vi "System3.vi"() -> ()   [LabVIEW 2015]
uses:
  <vilib>/addons/control/pid/NI_PID_autopid.lvlib
  <vilib>/DAQmx/write.llb/DAQmx Write (Analog DBL 1Chan 1Samp).vi
  <vilib>/DAQmx/read.llb/DAQmx Read (Analog 1D Wfm NChan NSamp).vi
  <vilib>/Analysis/NI_AALBase.lvlib
  <vilib>/Analysis/baseanly.llb/Mean (DBL).vi
  <vilib>/DAQmx/write.llb/DAQmx Write (Digital 1D Bool NChan 1Samp 1Line).vi
  Control 1.ctl
panel:
  in  "Open/Close (Green)":bool
  in  "Open/Close (Blue)":bool
  in  "Stop program":bool
  in  "On/Off":bool
  in  "Manual Control 2":bool
  in  "Voltage setting 2":dbl format="%#_13g"
  out "Voltage Reading(pressure) 2":dbl format="%#_13g"
  out "Pressure 2":dbl format="%#.3g"
  out "Pressure Chart 2":dbl(graph)
  in  "autotuning parameters 2":T1={"controller type"=1, "relay cycles"=3, "relay amplitude"=1.0, "control specification"=2, "PV noise level"=0.1} {"PV noise level" format="%.2f"; "control specification" items=["normal", "fast", "slow"]; "relay amplitude" format="%.2f"; "controller type" items=["PID", "PI", "P"]}
  in  "PID gains 2":T2={"proportional gain (Kc)"=1.0, "integral time (Ti, min)"=0.01, "derivative time (Td, min)"=0.0} {"derivative time (Td, min)" format="%.3f"; "integral time (Ti, min)" format="%.3f"; "proportional gain (Kc)" format="%.3f"}
  out "PID gains out 2":T2={"proportional gain (Kc)"=1.0, "integral time (Ti, min)"=0.01, "derivative time (Td, min)"=0.0} {"derivative time (Td, min)" format="%.3f"; "integral time (Ti, min)" format="%.3f"; "proportional gain (Kc)" format="%.3f"}
  in  "autotune? (F) 2":bool
  in  "reinitialize? (F) 2":bool
  in  "setpoint in Bar 2":dbl format="%#.5f"
  out "Control Value 2":dbl
  in  "Voltage setting":dbl format="%#_13g"
  in  "Manual Control":bool
  out "Control Value":dbl
  in  "setpoint in Bar":dbl format="%#.5f"
  in  "reinitialize? (F)":bool
  in  "autotune? (F)":bool
  out "PID gains out":T2={"proportional gain (Kc)"=1.0, "integral time (Ti, min)"=0.01, "derivative time (Td, min)"=0.0} {"derivative time (Td, min)" format="%.3f"; "integral time (Ti, min)" format="%.3f"; "proportional gain (Kc)" format="%.3f"}
  in  "PID gains":T2={"proportional gain (Kc)"=1.0, "integral time (Ti, min)"=0.01, "derivative time (Td, min)"=0.0} {"derivative time (Td, min)" format="%.3f"; "integral time (Ti, min)" format="%.3f"; "proportional gain (Kc)" format="%.3f"}
  in  "autotuning parameters":T1={"controller type"=1, "relay cycles"=3, "relay amplitude"=1.0, "control specification"=2, "PV noise level"=0.1} {"PV noise level" format="%.2f"; "control specification" items=["normal", "fast", "slow"]; "relay amplitude" format="%.2f"; "controller type" items=["PID", "PI", "P"]}
  out "Pressure Chart":dbl(graph)
  out "Pressure":dbl format="%#.3g"
  out "Voltage Reading(pressure)":dbl format="%#_13g"
  # "Pressure Vessel 2"
  # "Pressure Vessel 1"
  # "Readings"
  # "Controls"
  # "Readings"
  # "Controls"
  # "PID Settings"
  # "51.12139\n\n0.044676"
  # "Valves"
  # "Pump 3"
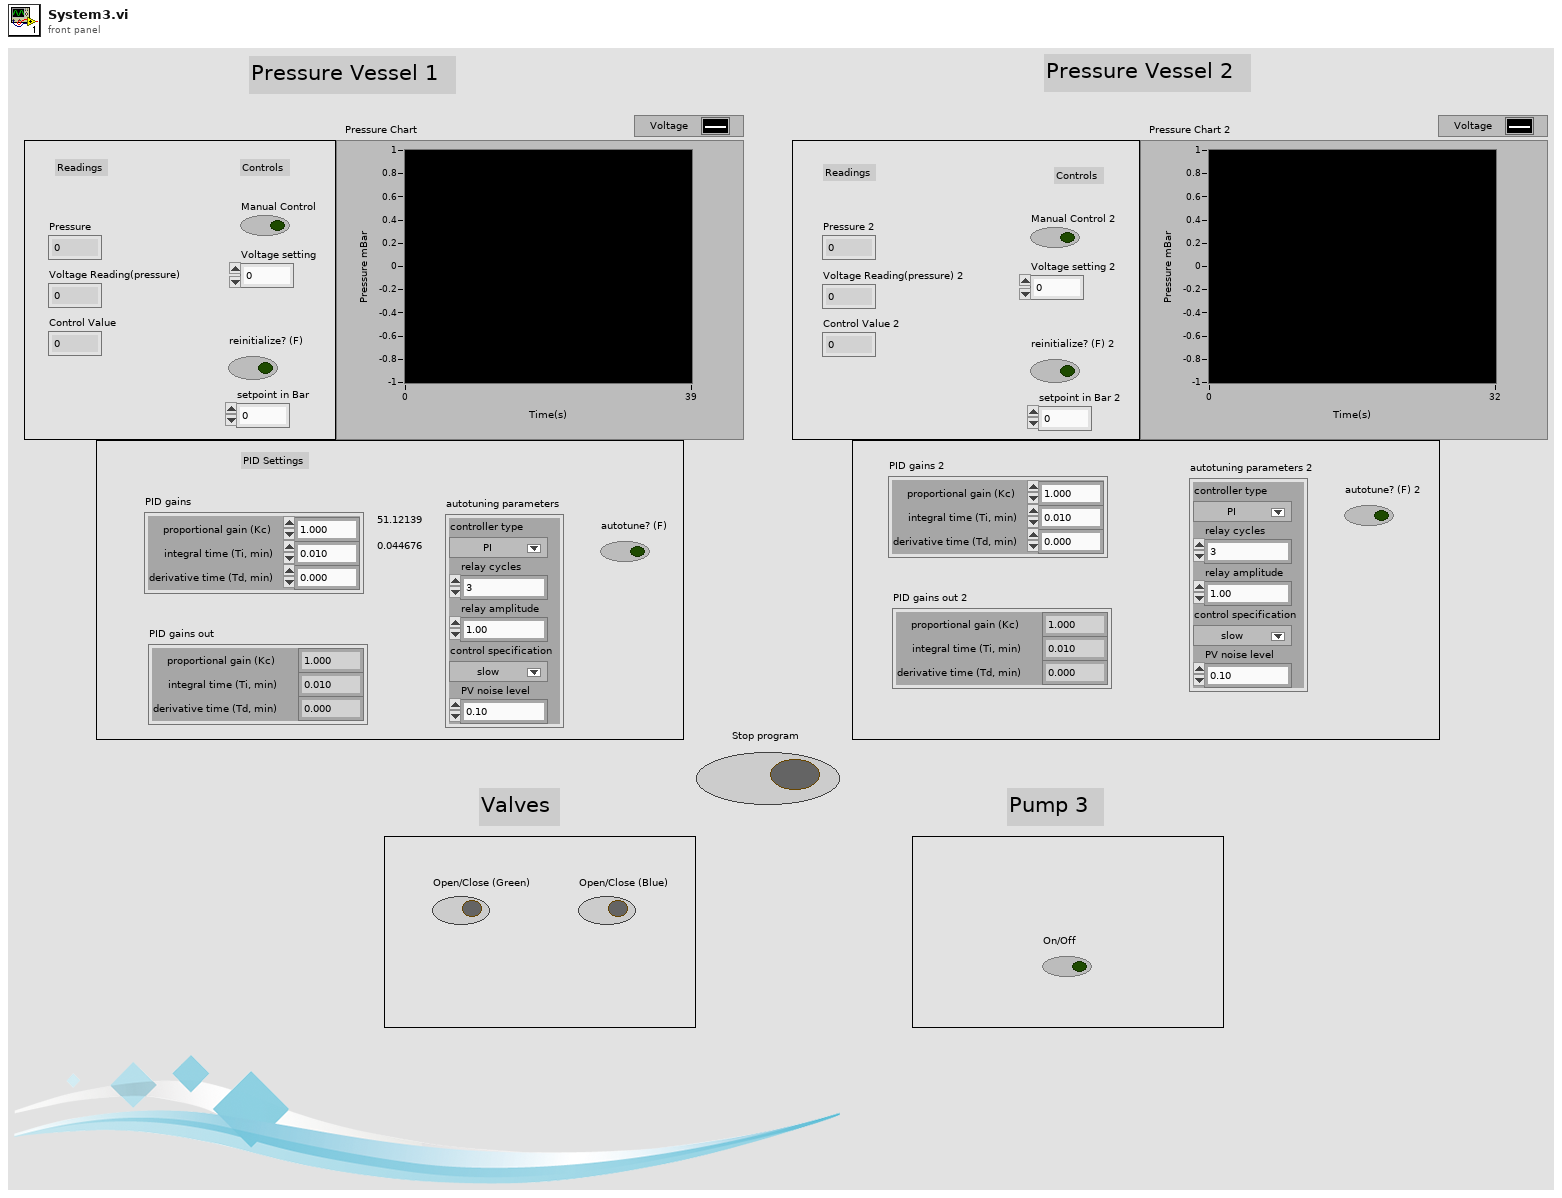
[diagram p1: front panel]
types:
  T1 = cluster{"controller type":u16, "relay cycles":i32, "relay amplitude":dbl, "control specification":u16, "PV noise level":dbl}
  T2 = cluster{"proportional gain (Kc)":dbl, "integral time (Ti, min)":dbl, "derivative time (Td, min)":dbl}
  T3 = typedef "Control 1.ctl" = refnum<k21>
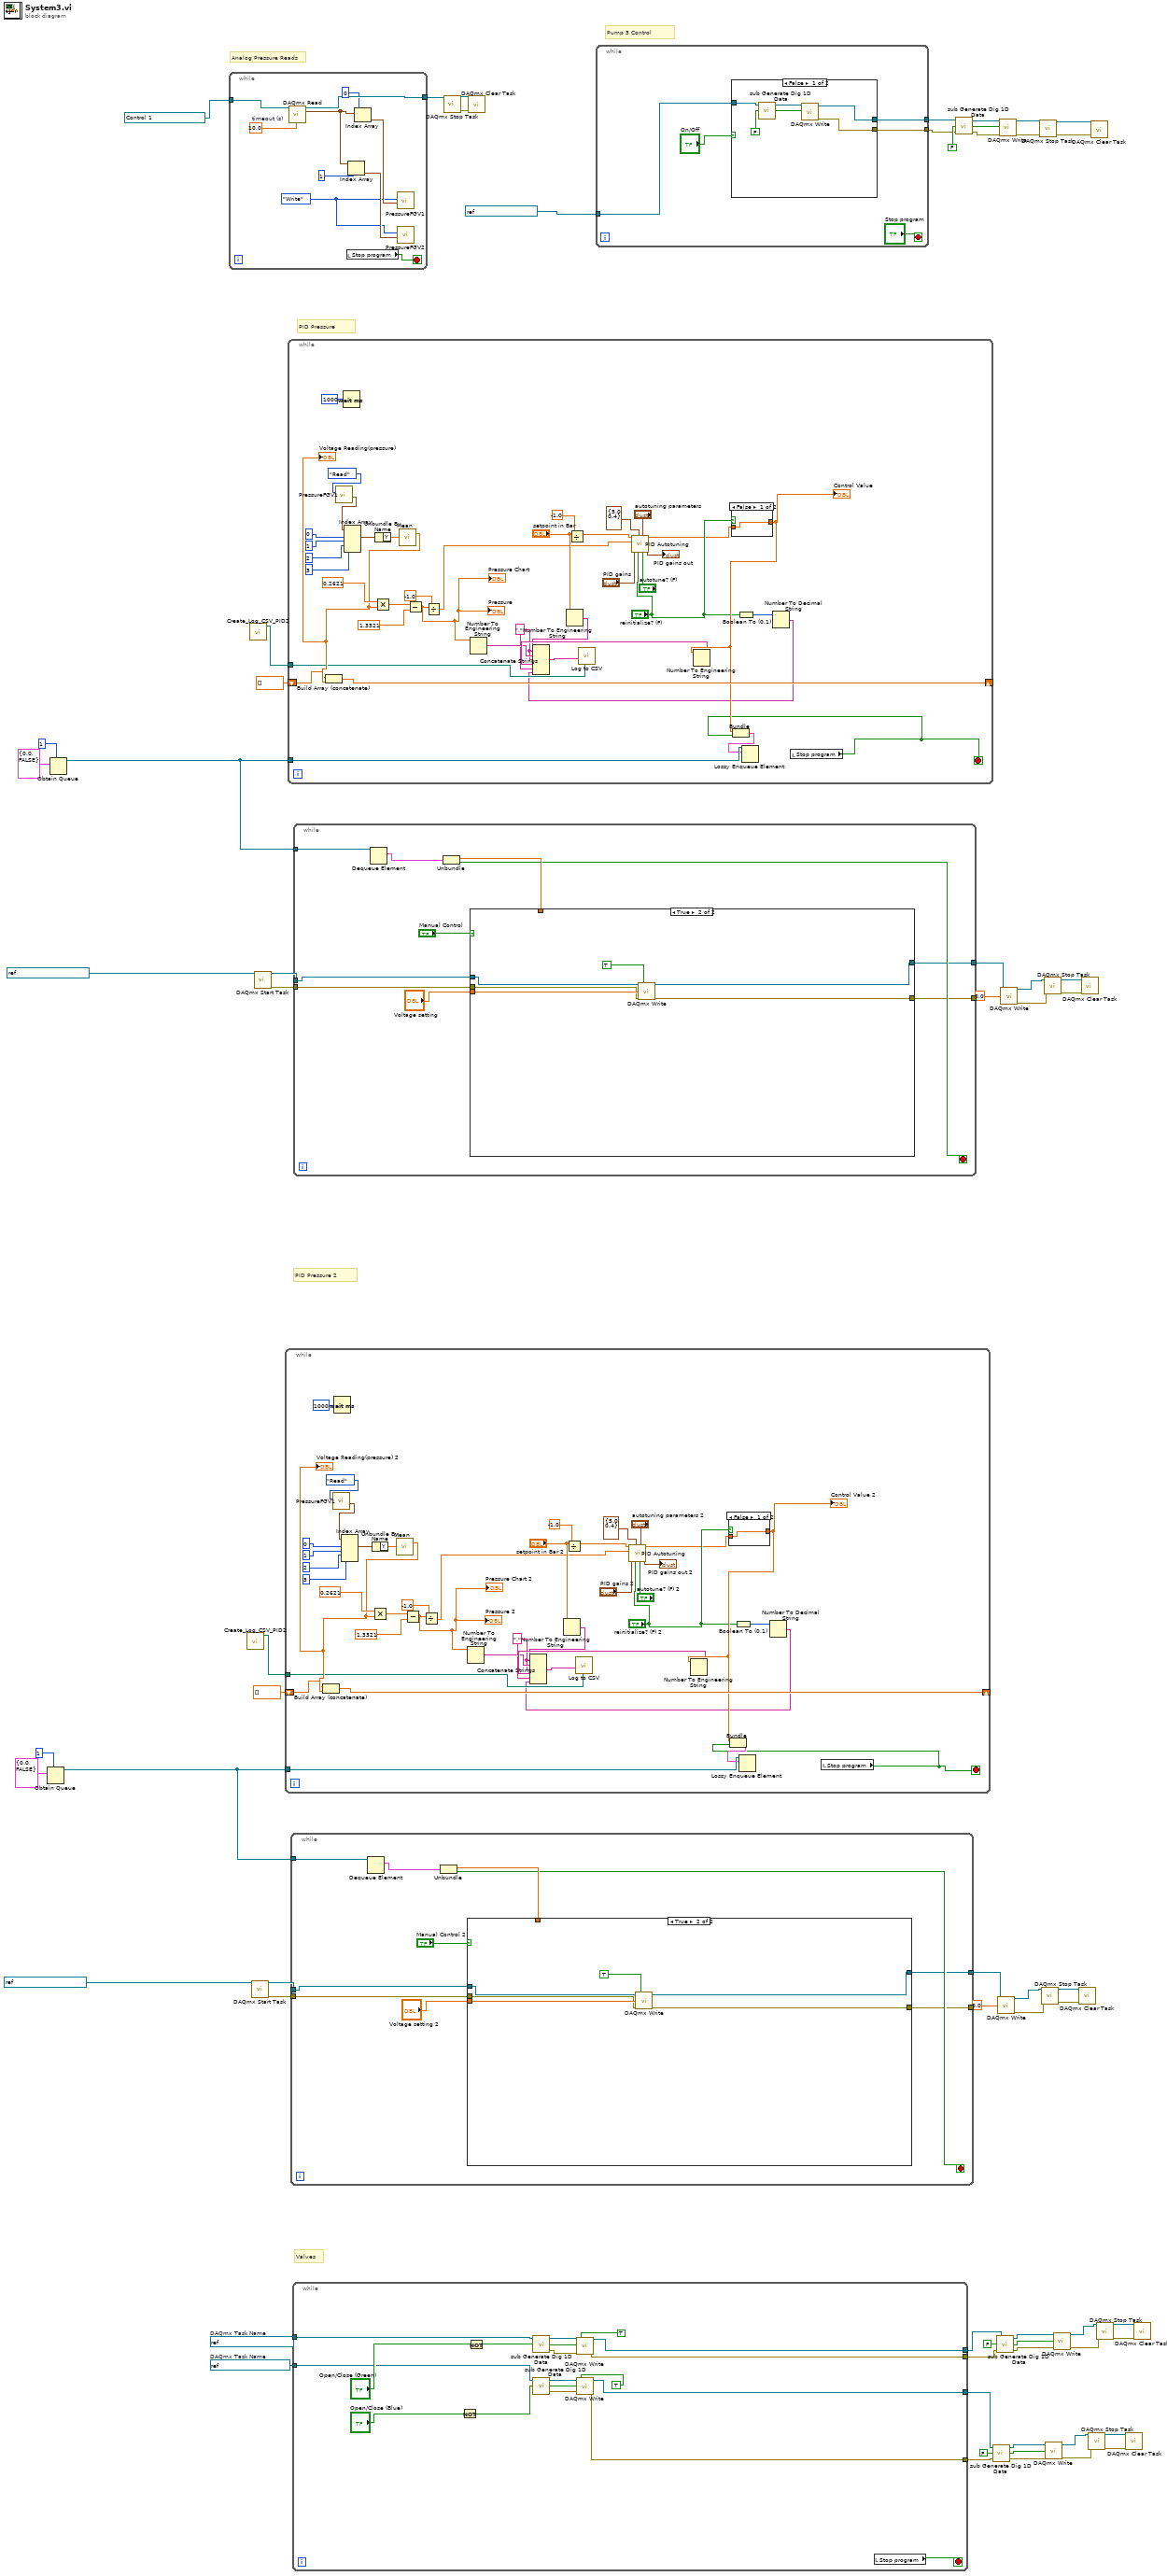
[diagram p0: block diagram]
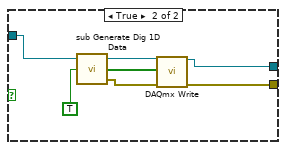
[diagram p2: hidden frame]
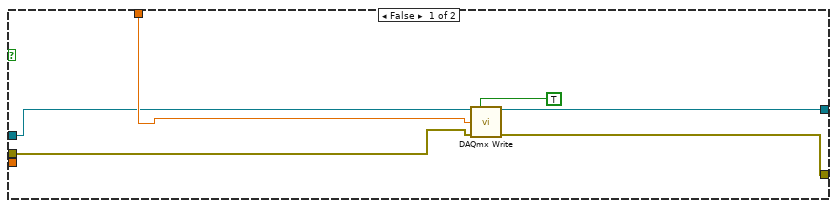
[diagram p3: hidden frame]
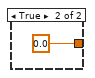
[diagram p4: hidden frame]
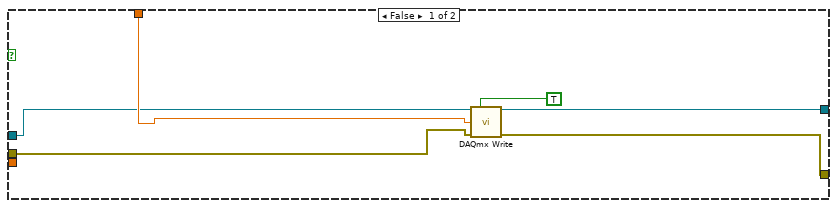
[diagram p5: hidden frame]
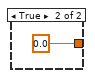
[diagram p6: hidden frame]
diagram:
  w25 = refnum<k21> "NewDigitalSystemBlue"  # DAQmx Task Name
  w26 = refnum<k21> "NewDigitalSystemGreen"  # DAQmx Task Name
  # "Analog Pressure Reads"
  # "Valves"
  # "Pump 3 Control"
  # "PID Pressure"
  # "PID Pressure 2"
  n1 = Obtain Queue(max queue size (-1, unlimited)=1, element data type=cluster{dbl, bool} {0.0, FALSE}) -> (queue out=w50:refnum<queue>)  [unwired: 3 in, 2 out]
  n2 = Obtain Queue(max queue size (-1, unlimited)=1, element data type=cluster{dbl, bool} {0.0, FALSE}) -> (queue out=w64:refnum<queue>)  [unwired: 3 in, 2 out]
  n3 = while {
    tunnel: T3 "New AnalogSystemAI0" -> [w73]
    tunnel: [w72] -> w1
    stop <- w75 stop-if-true
    w66 = enum16{"Write", "Read"}."Write" ("Command")
    w74 = 10.0  # timeout (s)
    n4 = call-poly <vilib>:"DAQmx Read.vi"("task/channels in"=w73, "timeout"=w74) -> ("task out"=w72:refnum<k21>, "data"=w69:waveform(dbl)[])  [unwired: 11 in, 1 out]
    n5 = local read "Stop program"() -> (w75:bool)
    n6 = Index Array(array=w69, index=1) -> (element=w67:waveform(dbl))
    n7 = Index Array(array=w69, index=0) -> (element=w70:waveform(dbl))
    n8 = call "PressureFGV1.vi"("Array"=w70, "Command"=w66) -> ()  [unwired: 9 in, 1 out]
    n9 = call "PressureFGV2.vi"("Array"=w67, "Command"=w66) -> ()  [unwired: 9 in, 1 out]
  }
  n10 = call "Create_Log_CSV_PID2.vi"() -> ("path"=w46:path)  [unwired: 11 in]
  n11 = call "Create_Log_CSV_PID2.vi"() -> ("path"=w60:path)  [unwired: 11 in]
  n12 = call <vilib>:"DAQmx Start Task.vi"("task/channels in"=refnum<k21> "NewAnalogSystemAO0") -> ("task out"=w45:refnum<k21>, "error out"=w44:errorcluster)  [unwired: 13 in]
  n13 = call <vilib>:"DAQmx Start Task.vi"("task/channels in"=refnum<k21> "NewAnalogSystemAO1") -> ("task out"=w59:refnum<k21>, "error out"=w58:errorcluster)  [unwired: 13 in]
  n14 = while {
    tunnel: w50 -> [w107]
    shift-right: [w98] -> _
    shift-left: dbl[] [] -> [w99]
    tunnel: w46 -> [w92]
    stop <- w79 stop-if-true
    w87 = ","
    n15 = call "PressureFGV1.vi"("Command"=enum16{"Write", "Read"}."Read") -> ("Array 2"=w76:waveform(dbl)[])  [unwired: 10 in]
    n16 = Wait (ms)(milliseconds to wait=u32 1000) -> ()  [unwired: 1 out]
    n17 = Index Array(array=w76, index #1=0 ("index"), index #2=1 ("index"), index #3=2 ("index"), index #4=3 ("index")) -> (element #1=w102:waveform(dbl))  [unwired: 3 out]
    n18 = Unbundle By Name(w102) -> ("Y"=w101:dbl[])
    n19 = call-poly <vilib>:"Mean.vi"("X"=w101) -> ("mean"=w100:dbl)  [unwired: 1 out]
    "Voltage Reading(pressure) 2" <- w100
    n20 = Build Array (concatenate)(w99, w100) -> (w98:dbl[])
    n21 = Multiply(x=0.2621, y=w100) -> (x*y=w114:dbl)
    n22 = Subtract(x=w114, y=1.3321) -> (x-y=w96:dbl)
    "Pressure 2" <- w96
    "Pressure Chart 2" <- w96
    n23 = Divide(x=w96, y=-1.0) -> (x/y=w84:dbl)
    n24 = Number To Engineering String(4:w96) -> (0:w91:string)  [unwired: 3 in]
    n25 = Number To Engineering String(4:"setpoint in Bar 2") -> (0:w90:string)  [unwired: 3 in]
    n26 = Divide(x="setpoint in Bar 2", y=-1.0) -> (x/y=w83:dbl)
    n27 = call <vilib>:"PID Autotuning.vi"("autotune? (F)"="autotune? (F) 2", "autotuning parameters"="autotuning parameters 2", "reinitialize? (F)"="reinitialize? (F) 2", "output range"=cluster{"output high":dbl, "output low":dbl} {"output high"=5.0, "output low"=0.4}, "PID gains"="PID gains 2", "process variable"=w84, "setpoint"=w83) -> ("PID gains out"=→"PID gains out 2":T2, "output"=w81:dbl)  [unwired: 1 in, 2 out]
    n28 = case shown="False" "reinitialize? (F) 2" {
      tunnel: [w116 0.0] -> w95
      tunnel: w81 -> [w116 _]
      frame False {
      }
      frame True {
      }
    }
    "Control Value 2" <- w95
    n29 = Number To Engineering String(4:w95) -> (0:w94:string)  [unwired: 3 in]
    n30 = Boolean To (0,1)(Boolean="reinitialize? (F) 2") -> (0, 1=w88:i16)
    n31 = Number To Decimal String(number=w88) -> (decimal integer string=w86:string)  [unwired: 1 in]
    n32 = Concatenate Strings(w90, w87, w91, w87, w94, w87, w86) -> (w93:string)
    n33 = call "Log to CSV.vi"("Data Str"=w93, "Path"=w92) -> ()  [unwired: 5 in, 1 out]
    n34 = local read "Stop program"() -> (w79:bool)
    n35 = Bundle("output"=w95, "Stop program"=w79) -> (w80:cluster{"output":dbl, "Stop program":bool})  [unwired: 1 in]
    n36 = Lossy Enqueue Element(queue=w107, element=w80) -> ()  [unwired: 1 in, 4 out]
  }
  n37 = while {
    tunnel: w64 -> [w149]
    shift-right: [w139] -> _
    shift-left: dbl[] [] -> [w140]
    tunnel: w60 -> [w133]
    stop <- w121 stop-if-true
    w128 = ","
    n38 = call "PressureFGV1.vi"("Command"=enum16{"Write", "Read"}."Read") -> ("Array 2"=w118:waveform(dbl)[])  [unwired: 10 in]
    n39 = Wait (ms)(milliseconds to wait=u32 1000) -> ()  [unwired: 1 out]
    n40 = Index Array(array=w118, index #1=0 ("index"), index #2=1 ("index"), index #3=2 ("index"), index #4=3 ("index")) -> (element #1=w143:waveform(dbl))  [unwired: 3 out]
    n41 = Unbundle By Name(w143) -> ("Y"=w142:dbl[])
    n42 = call-poly <vilib>:"Mean.vi"("X"=w142) -> ("mean"=w141:dbl)  [unwired: 1 out]
    "Voltage Reading(pressure)" <- w141
    n43 = Build Array (concatenate)(w140, w141) -> (w139:dbl[])
    n44 = Multiply(x=0.2621, y=w141) -> (x*y=w156:dbl)
    n45 = Subtract(x=w156, y=1.3321) -> (x-y=w137:dbl)
    "Pressure" <- w137
    "Pressure Chart" <- w137
    n46 = Divide(x=w137, y=-1.0) -> (x/y=w125:dbl)
    n47 = Number To Engineering String(4:w137) -> (0:w132:string)  [unwired: 3 in]
    n48 = Number To Engineering String(4:"setpoint in Bar") -> (0:w131:string)  [unwired: 3 in]
    n49 = Divide(x="setpoint in Bar", y=-1.0) -> (x/y=w124:dbl)
    n50 = call <vilib>:"PID Autotuning.vi"("autotune? (F)"="autotune? (F)", "autotuning parameters"="autotuning parameters", "reinitialize? (F)"="reinitialize? (F)", "output range"=cluster{"output high":dbl, "output low":dbl} {"output high"=5.0, "output low"=0.4}, "PID gains"="PID gains", "process variable"=w125, "setpoint"=w124) -> ("PID gains out"=→"PID gains out":T2, "output"=w122:dbl)  [unwired: 1 in, 2 out]
    n51 = case shown="False" "reinitialize? (F)" {
      tunnel: [w158 0.0] -> w136
      tunnel: w122 -> [w158 _]
      frame False {
      }
      frame True {
      }
    }
    "Control Value" <- w136
    n52 = Number To Engineering String(4:w136) -> (0:w135:string)  [unwired: 3 in]
    n53 = Boolean To (0,1)(Boolean="reinitialize? (F)") -> (0, 1=w129:i16)
    n54 = Number To Decimal String(number=w129) -> (decimal integer string=w127:string)  [unwired: 1 in]
    n55 = Concatenate Strings(w131, w128, w132, w128, w135, w128, w127) -> (w134:string)
    n56 = call "Log to CSV.vi"("Data Str"=w134, "Path"=w133) -> ()  [unwired: 5 in, 1 out]
    n57 = local read "Stop program"() -> (w121:bool)
    n58 = Bundle("output"=w136, "Stop program"=w121) -> (w148:cluster{"output":dbl, "Stop program":bool})  [unwired: 1 in]
    n59 = Lossy Enqueue Element(queue=w149, element=w148) -> ()  [unwired: 1 in, 4 out]
  }
  n60 = while {
    tunnel: w50 -> [w169]
    tunnel: w45 -> [w167]
    tunnel: [w162] -> w42
    tunnel: w44 -> [w161]
    tunnel: [w160] -> _
    stop <- w163 stop-if-true
    n61 = Dequeue Element(queue=w169) -> (element=w166:cluster{dbl, bool})  [unwired: 2 in, 3 out]
    n62 = Unbundle(w166) -> (w165:dbl, w163:bool)
    n63 = case shown="True" "Manual Control 2" {
      tunnel: w167 -> [w173 w180]
      tunnel: w165 -> [w174 _]
      tunnel: "Voltage setting 2" -> [_ w179]
      tunnel: [w172 w178] -> w162
      tunnel: w161 -> [w171 w177]
      tunnel: [w170 w176] -> w160
      frame False {
        n64 = call-poly <vilib>:"DAQmx Write.vi"("task/channels in"=w173, "auto start"=TRUE, "data"=w174, "error in"=w171) -> ("task out"=w172:refnum<k21>, "error out"=w170:errorcluster)  [unwired: 9 in, 1 out]
      }
      frame True {
        n65 = call-poly <vilib>:"DAQmx Write.vi"("task/channels in"=w180, "auto start"=TRUE, "data"=w179, "error in"=w177) -> ("task out"=w178:refnum<k21>, "error out"=w176:errorcluster)  [unwired: 9 in, 1 out]
      }
    }
  }
  n66 = while {
    tunnel: w26 -> [w190]
    tunnel: w25 -> [w189]
    tunnel: [w188] -> w15
    tunnel: [w187] -> w11
    tunnel: [w184] -> w8
    tunnel: [w183] -> w6
    stop <- w182 stop-if-true
    n67 = Not(x="Open/Close (Blue)") -> (.not. x?=w200:bool)
    n68 = Not(x="Open/Close (Green)") -> (.not. x?=w199:bool)
    n69 = call <vilib>:"sub Generate Dig 1D Data.vi"("initial value"=w199, "task in"=w190) -> ("error out"=w186:errorcluster, "Data"=w197:bool[], "task out"=w194:refnum<k21>)  [unwired: 1 in]
    n70 = call <vilib>:"sub Generate Dig 1D Data.vi"("initial value"=w200, "task in"=w189) -> ("error out"=w185:errorcluster, "Data"=w196:bool[], "task out"=w195:refnum<k21>)  [unwired: 1 in]
    n71 = call-poly <vilib>:"DAQmx Write.vi"("task/channels in"=w194, "auto start"=TRUE, "data"=w197, "error in"=w186) -> ("task out"=w188:refnum<k21>, "error out"=w184:errorcluster)  [unwired: 9 in, 1 out]
    n72 = call-poly <vilib>:"DAQmx Write.vi"("task/channels in"=w195, "auto start"=TRUE, "data"=w196, "error in"=w185) -> ("task out"=w187:refnum<k21>, "error out"=w183:errorcluster)  [unwired: 9 in, 1 out]
    n73 = local read "Stop program"() -> (w182:bool)
  }
  n74 = while {
    tunnel: w64 -> [w210]
    tunnel: w59 -> [w208]
    tunnel: [w203] -> w56
    tunnel: w58 -> [w202]
    tunnel: [w201] -> _
    stop <- w204 stop-if-true
    n75 = Dequeue Element(queue=w210) -> (element=w207:cluster{dbl, bool})  [unwired: 2 in, 3 out]
    n76 = Unbundle(w207) -> (w206:dbl, w204:bool)
    n77 = case shown="True" "Manual Control" {
      tunnel: w208 -> [w214 w221]
      tunnel: w206 -> [w215 _]
      tunnel: "Voltage setting" -> [_ w220]
      tunnel: [w213 w219] -> w203
      tunnel: w202 -> [w212 w218]
      tunnel: [w211 w217] -> w201
      frame False {
        n78 = call-poly <vilib>:"DAQmx Write.vi"("task/channels in"=w214, "auto start"=TRUE, "data"=w215, "error in"=w212) -> ("task out"=w213:refnum<k21>, "error out"=w211:errorcluster)  [unwired: 9 in, 1 out]
      }
      frame True {
        n79 = call-poly <vilib>:"DAQmx Write.vi"("task/channels in"=w221, "auto start"=TRUE, "data"=w220, "error in"=w218) -> ("task out"=w219:refnum<k21>, "error out"=w217:errorcluster)  [unwired: 9 in, 1 out]
      }
    }
  }
  n80 = call <vilib>:"DAQmx Stop Task.vi"("task/channels in"=w1) -> ("task out"=w3:refnum<k21>, "error out"=w2:errorcluster)  [unwired: 13 in]
  n81 = call <vilib>:"DAQmx Clear Task.vi"("task in"=w3, "error in"=w2) -> ()  [unwired: 13 in, 1 out]
  n82 = while {
    tunnel: refnum<k21> "NewDigSystemP0L2" -> [w226]
    tunnel: [w225] -> w30
    tunnel: [w224] -> w29
    stop <- "Stop program" stop-if-true
    n83 = case shown="False" "On/Off" {
      tunnel: w226 -> [w233 w237]
      tunnel: [w229 w236] -> w225
      tunnel: [w228 w234] -> w224
      frame False {
        n84 = call <vilib>:"sub Generate Dig 1D Data.vi"("initial value"=FALSE, "task in"=w233) -> ("Data"=w231:bool[], "task out"=w232:refnum<k21>)  [unwired: 1 in, 1 out]
        n85 = call-poly <vilib>:"DAQmx Write.vi"("task/channels in"=w232, "data"=w231) -> ("task out"=w229:refnum<k21>, "error out"=w228:errorcluster)  [unwired: 11 in, 1 out]
      }
      frame True {
        n86 = call <vilib>:"sub Generate Dig 1D Data.vi"("initial value"=TRUE, "task in"=w237) -> ("error out"=w235:errorcluster, "Data"=w239:bool[], "task out"=w238:refnum<k21>)  [unwired: 1 in]
        n87 = call-poly <vilib>:"DAQmx Write.vi"("task/channels in"=w238, "data"=w239, "error in"=w235) -> ("task out"=w236:refnum<k21>, "error out"=w234:errorcluster)  [unwired: 10 in, 1 out]
      }
    }
  }
  n88 = call <vilib>:"sub Generate Dig 1D Data.vi"("error in"=w29, "initial value"=FALSE, "task in"=w30) -> ("error out"=w34:errorcluster, "Data"=w32:bool[], "task out"=w33:refnum<k21>)
  n89 = call <vilib>:"sub Generate Dig 1D Data.vi"("error in"=w6, "initial value"=FALSE, "task in"=w11) -> ("error out"=w5:errorcluster, "Data"=w10:bool[], "task out"=w12:refnum<k21>)
  n90 = call <vilib>:"sub Generate Dig 1D Data.vi"("error in"=w8, "initial value"=FALSE, "task in"=w15) -> ("error out"=w7:errorcluster, "Data"=w9:bool[], "task out"=w16:refnum<k21>)
  n91 = call-poly <vilib>:"DAQmx Write.vi"("task/channels in"=w42, "data"=0.0) -> ("task out"=w41:refnum<k21>, "error out"=w40:errorcluster)  [unwired: 11 in, 1 out]
  n92 = call-poly <vilib>:"DAQmx Write.vi"("task/channels in"=w33, "data"=w32, "error in"=w34) -> ("task out"=w28:refnum<k21>, "error out"=w27:errorcluster)  [unwired: 10 in, 1 out]
  n93 = call-poly <vilib>:"DAQmx Write.vi"("task/channels in"=w56, "data"=0.0) -> ("task out"=w55:refnum<k21>, "error out"=w54:errorcluster)  [unwired: 11 in, 1 out]
  n94 = call <vilib>:"DAQmx Stop Task.vi"("task/channels in"=w28, "error in"=w27) -> ("task out"=w36:refnum<k21>, "error out"=w35:errorcluster)  [unwired: 12 in]
  n95 = call <vilib>:"DAQmx Stop Task.vi"("task/channels in"=w41, "error in"=w40) -> ("task out"=w43:refnum<k21>, "error out"=w39:errorcluster)  [unwired: 12 in]
  n96 = call <vilib>:"DAQmx Stop Task.vi"("task/channels in"=w55, "error in"=w54) -> ("task out"=w57:refnum<k21>, "error out"=w53:errorcluster)  [unwired: 12 in]
  n97 = call-poly <vilib>:"DAQmx Write.vi"("task/channels in"=w12, "data"=w10, "error in"=w5) -> ("task out"=w19:refnum<k21>, "error out"=w18:errorcluster)  [unwired: 10 in, 1 out]
  n98 = call-poly <vilib>:"DAQmx Write.vi"("task/channels in"=w16, "data"=w9, "error in"=w7) -> ("task out"=w22:refnum<k21>, "error out"=w23:errorcluster)  [unwired: 10 in, 1 out]
  n99 = call <vilib>:"DAQmx Clear Task.vi"("task in"=w43, "error in"=w39) -> ()  [unwired: 13 in, 1 out]
  n100 = call <vilib>:"DAQmx Clear Task.vi"("task in"=w57, "error in"=w53) -> ()  [unwired: 13 in, 1 out]
  n101 = call <vilib>:"DAQmx Stop Task.vi"("task/channels in"=w19, "error in"=w18) -> ("task out"=w20:refnum<k21>, "error out"=w17:errorcluster)  [unwired: 12 in]
  n102 = call <vilib>:"DAQmx Clear Task.vi"("task in"=w36, "error in"=w35) -> ()  [unwired: 13 in, 1 out]
  n103 = call <vilib>:"DAQmx Stop Task.vi"("task/channels in"=w22, "error in"=w23) -> ("task out"=w21:refnum<k21>, "error out"=w24:errorcluster)  [unwired: 12 in]
  n104 = call <vilib>:"DAQmx Clear Task.vi"("task in"=w20, "error in"=w17) -> ()  [unwired: 13 in, 1 out]
  n105 = call <vilib>:"DAQmx Clear Task.vi"("task in"=w21, "error in"=w24) -> ()  [unwired: 13 in, 1 out]
